vi "Quad Ctr.vi"() -> ()   [LabVIEW 2015]
doc: "This VI uses the quadrature encoder hardware on the evaluation board to count pulses on the encoder. The 8-bit count is used to display the current count position of the encoder. Use the reset button to reinitialize the quadrature encoder count to zero."
uses:
  <vilib>/eio/EIONode/EIONode.xnode
  <vilib>/Platform/TimedLoop/XDataNode/XDataNode.xnode
  <vilib>/Platform/TimedLoop/XDataNode/nitl_modes.ctl
  <vilib>/Platform/TimedLoop/XDataNode/XDNodeRunTimeDep.lvlib
  <vilib>/Platform/TimedLoop/XDataNode/wakeup.ctl
  <vilib>/Platform/TimedLoop/XDataNode/timing_clust.ctl
  <vilib>/rvi/eio/common/nirviEmuTemplateMethod_errors.vi
panel:
  out "8-bit Count":u8
  in  "stop":bool
  in  "Reset":bool
  # "This VI uses the quadrature encoder hardware on the evaluation board to count pulses on the encoder.  The 8-bit count is used to display the current count position of the encoder.  Use the reset button to reinitialize the quadrature encoder count to zero."
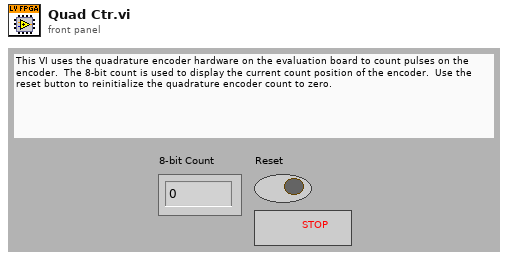
[diagram p1: front panel]
types:
  T1 = typedef "XDNodeRunTimeDep.lvlib/timing_clust.ctl" = cluster{"Expected End [f-1]":u64, "Actual End [f-1]":u64, "Finished Late? [f-1]":bool, "Expected End [i-1]":u64, "Actual End [i-1]":u64, "Finished Late? [i-1]":bool, "Expected Start [i]":u64, "Actual Start [i]":u64, "Expected Start [f]":u64, "Actual Start [f]":u64, "Source Name":string, "Structure Name":string, "Period":i64, "Deadline":i64, "Offset":i64, "Start":i64, "Priority":i32, "Timeout":i32, "Mode":T2, "Wakeup Reason":T3, "Error":errorcluster, "Source Type":string, "Secondary Source Type":string, "Global End Time":u64, "Global Start Time":u64, "Frame Duration":u64, "Iteration Duration":u64, "Assigned CPU":i32, "I/O Scan Engine Mode":u32}
  T2 = typedef "XDNodeRunTimeDep.lvlib/nitl_modes.ctl" = enum32{"No Change", "Process missed periods, maintain original phase", "Discard missed periods, maintain original phase", "Process missed periods, ignore original phase", "Discard missed periods, ignore original phase"}
  T3 = typedef "XDNodeRunTimeDep.lvlib/wakeup.ctl" = enum32{"Normal", "Aborted", "Asynchronous wakeup", "Timing source error", "Timed loop error", "Timeout"}
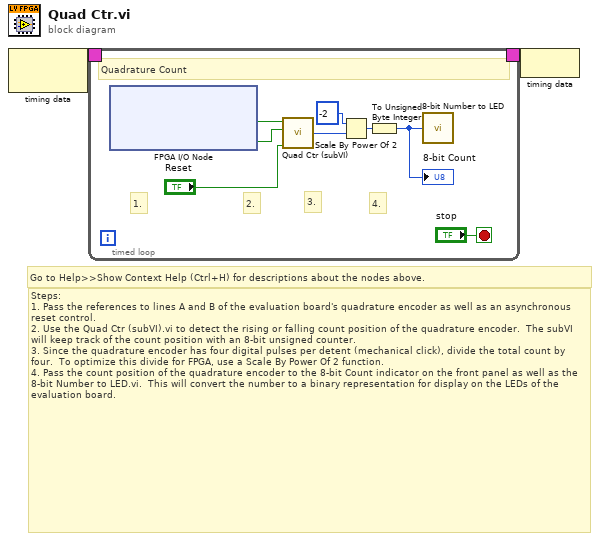
[diagram p0: block diagram]
diagram:
  # "Go to Help>>Show Context Help (Ctrl+H) for descriptions about the nodes above."
  # "Steps:\n1. Pass the references to lines A and B of the evaluation board's quadrature encoder as well as an asynchronous reset control.\n2. Use the Quad Ctr (subVI).vi to detect the rising or falling count position of the quadrature encoder.  The subVI will keep track of the count position with an 8-bit unsigned counter.\n3. Since the quadrature encoder has four digital pulses per detent (mechanical click), divide the total count by four.  To optimize this divide for FPGA, use a Scale By Power Of 2 function.\n4. Pass the count position of the quadrature encoder to the 8-bit Count indicator on the front panel as well as the 8-bit Number to LED.vi.  This will convert the number to a binary representation for display on the LEDs of the evaluation board."
  n1 = node-c288() -> (w2:T1)  [unwired: 1 out]
  n2 = timed-loop {
    timing: w2 -> [_]
    timing-out: [_] -> w1
    stop <- "stop" stop-if-true
    # "4."
    # "3."
    # "2."
    # "1."
    # "Quadrature Count"
    n3 = xnode "FPGA I/O Node"() -> ("ENCODER CH.A"=w10:bool, "ENCODER CH.B"=w7:bool)  [unwired: 2 in, 2 out]
    n4 = call "Quad Ctr (subVI).vi"("Reset"="Reset", "Input B"=w7, "Input A"=w10) -> ("16-bit Count"=w5:u16)  [unwired: 1 out]
    n5 = Scale By Power Of 2(n=-2, x=w5) -> (x*2^n=w4:u16)
    n6 = To Unsigned Byte Integer(number=w4) -> (unsigned 8bit integer=w3:u8)
    "8-bit Count" <- w3
    n7 = call "8-bit Number to LED.vi"("8-bit Unsigned Number"=w3) -> ()  [unwired: 1 out]
  }
  n8 = node-c288(w1) -> ()
